vi "Run.vi"(8 "error in (no error)":errorcluster, 11 "WeatherSensor in":refnum<class "WeatherSensor.lvclass">) -> (0 "error out":errorcluster, 3 "WeatherSensor out":refnum<class "WeatherSensor.lvclass">)   [LabVIEW 2018, in "WeatherSensor.lvclass"]
uses:
  WeatherSensor.lvclass
  C:/Users/observer/Desktop/Sparc4GUI/Versao ZeroMQ/SPARC4_GUI - Desenv/Device/Device.lvclass
  Device/Device.lvclass/Device.ctl
  WeatherSensor.lvclass/WeatherSensor.ctl
  Device/Device.lvclass
  StateMachine/State Machine.lvclass
panel:
  out "WS erro":errorcluster
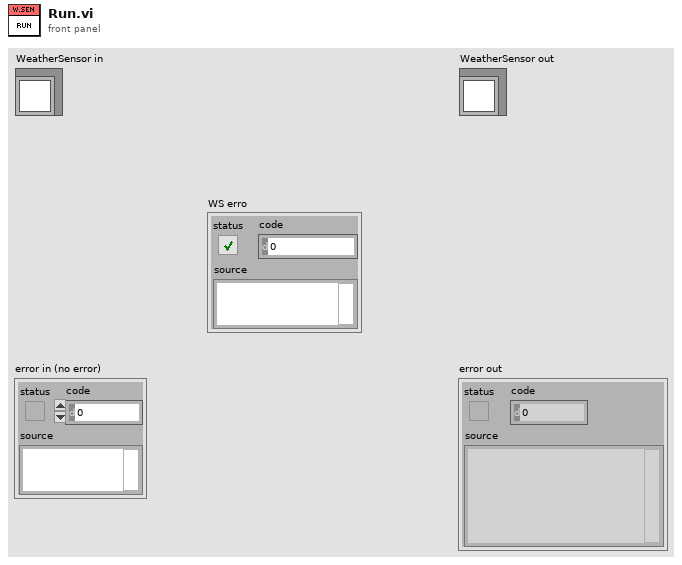
[diagram p1: front panel]
types:
  T1 = cluster{"broker":string, "version":string, "date":string, "hour":string, "outHumidity":string, "inHumidity":string, "inTemp":string, "outTemp":string, "windSpeed":string, "windDirection":string, "pressure":string, "dewOut":string, "dewIn":string, "leaf":string, "rain":string, "windChill":string}
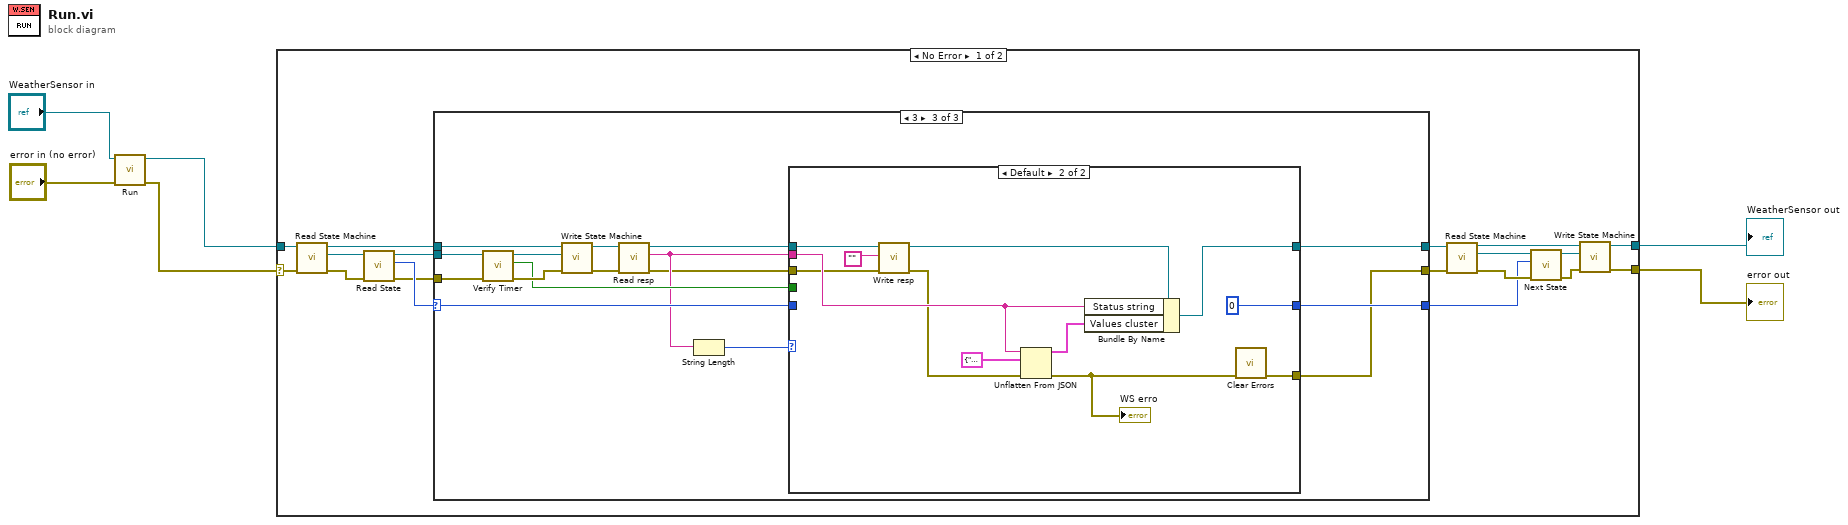
[diagram p0: block diagram]
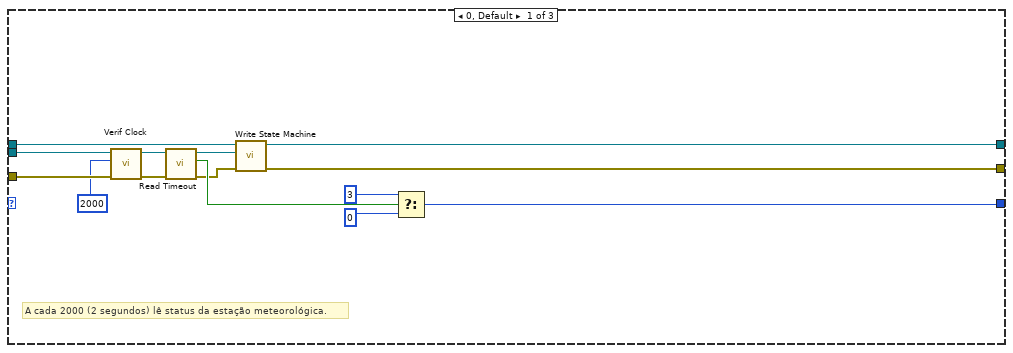
[diagram p2: hidden frame]
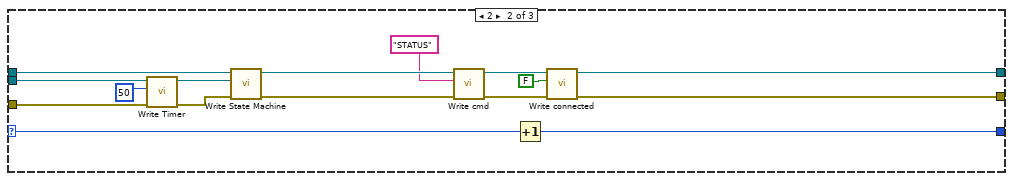
[diagram p3: hidden frame]
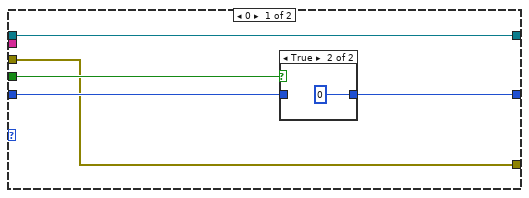
[diagram p4: hidden frame]
diagram:
  n1 = call-parent "Run.vi"("error in (no error)"="error in (no error)", "Device in"="WeatherSensor in") -> ("error out"=w3:errorcluster, "Device out"=w4:refnum<class "WeatherSensor.lvclass">)  [unwired: 8 in]
  n2 = case shown="No Error" w3 {
    selector: w3 -> [w23 w91]
    tunnel: [w15 w91] -> w2
    tunnel: w4 -> [w24 w90]
    tunnel: [w14 w90] -> w1
    frame No Error {
      n3 = call-dynamic "Read State Machine.vi"("error in (no error)"=w23, "Device in"=w24) -> ("error out"=w21:errorcluster, "State Machine.lvclass"=w22:refnum<class "State Machine.lvclass">, "Device out"=w12:refnum<class "WeatherSensor.lvclass">)  [unwired: 7 in]
      n4 = call-dynamic "Read State.vi"("error in (no error)"=w21, "State Machine in"=w22) -> ("error out"=w11:errorcluster, "State"=w13:i32, "State Machine out"=w7:refnum<class "State Machine.lvclass">)  [unwired: 7 in]
      n5 = case shown="3" w13 {
        selector: w13 -> [_ w54 w60]
        tunnel: w12 -> [w30 w50 w65]
        tunnel: w11 -> [w33 w48 w63]
        tunnel: [w26 w41 w55] -> w10
        tunnel: [w27 w43 w69] -> w9
        tunnel: [w38 w53 w68] -> w8
        tunnel: w7 -> [w32 w52 w67]
        frame 0, Default {
          # "A cada 2000 (2 segundos) lê status da estação meteorológica."
          n6 = call-dynamic "Verif Clock.vi"("error in (no error)"=w33, "period (ms)"=u32 2000 ("period"), "State Machine in"=w32) -> ("error out"=w34:errorcluster, "State Machine out"=w31:refnum<class "State Machine.lvclass">)  [unwired: 6 in, 1 out]
          n7 = call-dynamic "Read Timeout.vi"("error in (no error)"=w34, "State Machine in"=w31) -> ("error out"=w28:errorcluster, "Timeout"=w35:bool, "State Machine out"=w29:refnum<class "State Machine.lvclass">)  [unwired: 7 in]
          n8 = call-dynamic "Write State Machine.vi"("error in (no error)"=w28, "State Machine.lvclass"=w29, "Device in"=w30) -> ("error out"=w26:errorcluster, "Device out"=w27:refnum<class "WeatherSensor.lvclass">)  [unwired: 7 in]
          n9 = Select(t=3 ("State"), s=w35, f=0 ("State")) -> (s? t:f=w38:i32)
        }
        frame 2 {
          n10 = call-dynamic "Write Timer.vi"("error in (no error)"=w48, "Timer"=u32 50, "State Machine in"=w52) -> ("error out"=w47:errorcluster, "State Machine out"=w46:refnum<class "State Machine.lvclass">)  [unwired: 7 in]
          n11 = call-dynamic "Write State Machine.vi"("error in (no error)"=w47, "State Machine.lvclass"=w46, "Device in"=w50) -> ("error out"=w45:errorcluster, "Device out"=w49:refnum<class "WeatherSensor.lvclass">)  [unwired: 7 in]
          n12 = call-dynamic "Write cmd.vi"("error in (no error)"=w45, "cmd"="STATUS", "Device in"=w49) -> ("error out"=w42:errorcluster, "Device out"=w44:refnum<class "WeatherSensor.lvclass">)  [unwired: 7 in]
          n13 = Increment(x=w54) -> (x+1=w53:i32)
          n14 = call "Write connected.vi"("error in (no error)"=w42, "connected"=FALSE, "Device in"=w44) -> ("error out"=w41:errorcluster, "Device out"=w43:refnum<class "WeatherSensor.lvclass">)  [unwired: 7 in]
        }
        frame 3 {
          n15 = call "Verify Timer.vi"("error in (no error)"=w63, "State Machine in"=w67) -> ("error out"=w64:errorcluster, "timeout"=w59:bool, "State Machine out"=w66:refnum<class "State Machine.lvclass">)  [unwired: 7 in]
          n16 = call-dynamic "Write State Machine.vi"("error in (no error)"=w64, "State Machine.lvclass"=w66, "Device in"=w65) -> ("error out"=w61:errorcluster, "Device out"=w62:refnum<class "WeatherSensor.lvclass">)  [unwired: 7 in]
          n17 = call-dynamic "Read resp.vi"("error in (no error)"=w61, "Device in"=w62) -> ("error out"=w56:errorcluster, "resp"=w57:string, "Device out"=w70:refnum<class "WeatherSensor.lvclass">)  [unwired: 7 in]
          n18 = String Length(string=w57) -> (length=w58:i32)
          n19 = case shown="Default" w58 {
            tunnel: w70 -> [w75 w89]
            tunnel: [w75 w82] -> w69
            tunnel: [w73 0 ("State")] -> w68
            tunnel: w60 -> [w74 _]
            tunnel: w59 -> [w72 _]
            tunnel: w57 -> [_ w86]
            tunnel: w56 -> [w71 w84]
            tunnel: [w71 w78] -> w55
            frame 0 {
              n20 = case shown="True" w72 {
                tunnel: w74 -> [w76 _]
                tunnel: [w76 0 ("State")] -> w73
                frame False {
                }
                frame True {
                }
              }
            }
            frame Default {
              n21 = call-dynamic "Write resp.vi"("error in (no error)"=w84, "resp"="", "Device in"=w89) -> ("error out"=w83:errorcluster, "Device out"=w88:refnum<class "WeatherSensor.lvclass">)  [unwired: 7 in]
              n22 = Unflatten From JSON(JSON string=w86, type and defaults=T1 {"broker"="", "version"="", "date"="", "hour"="", "outHumidity"="", "inHumidity"="", "inTemp"="", "outTemp"="", "windSpeed"="", "windDirection"="", "pressure"="", "dewOut"="", "dewIn"="", "leaf"="", "rain"="", "windChill"=""} ("Values cluster"), error in (no error)=w83) -> (value=w81:T1, error out=w79:errorcluster)  [unwired: 4 in]
              "WS erro" <- w79
              n23 = Bundle By Name(cluster=w88, "Status string"=w86, "Values cluster"=w81) -> (w82:refnum<class "WeatherSensor.lvclass">)
              n24 = call <vilib>:"Clear Errors.vi"("error in (no error)"=w79) -> ("error out"=w78:errorcluster)  [unwired: 5 in, 1 out]
            }
          }
        }
      }
      n25 = call-dynamic "Read State Machine.vi"("error in (no error)"=w10, "Device in"=w9) -> ("error out"=w17:errorcluster, "State Machine.lvclass"=w19:refnum<class "State Machine.lvclass">, "Device out"=w18:refnum<class "WeatherSensor.lvclass">)  [unwired: 7 in]
      n26 = call "Next State.vi"("error in (no error)"=w17, "New_State"=w8, "State Machine in"=w19) -> ("error out"=w16:errorcluster, "State Machine out"=w20:refnum<class "State Machine.lvclass">)  [unwired: 7 in]
      n27 = call-dynamic "Write State Machine.vi"("error in (no error)"=w16, "State Machine.lvclass"=w20, "Device in"=w18) -> ("error out"=w15:errorcluster, "Device out"=w14:refnum<class "WeatherSensor.lvclass">)  [unwired: 7 in]
    }
    frame Error {
    }
  }
  "error out" <- w2
  "WeatherSensor out" <- w1
